vi "Simple TCP - Client.vi"() -> ()   [LabVIEW 2015]
doc: "Demonstrates how to open a connection to an TCP server, read the data being sent, and display the data on a chart. This VI is designed to stop if the TCP connection is terminated."
uses:
  <vilib>/Platform/TimedLoop/XDataNode/timing_clust.ctl
  <vilib>/Platform/TimedLoop/XDataNode/nitl_modes.ctl
  <vilib>/Platform/TimedLoop/XDataNode/wakeup.ctl
  <vilib>/platform/TimedLoop/XDataNode/XDataNode.xnode
  <vilib>/Platform/TimedLoop/XDataNode/XDNodeRunTimeDep.lvlib
panel:
  out "Counter":i32
  out "Time":u32
  out "value":T1
  in  "Server Closed":string="The server VI closed the connection."
  in  "Stop":bool
  # "Overview: Demonstrates the use of the TCP functions to connect to a TCP server VI and receive data.\nInstructions:\n1. Ensure Simple TCP - Server.vi is already running.\n2. Run the VI.\n3. Click Stop to stop the VI. Note that if you stop the server VI, this VI will stop automatically."
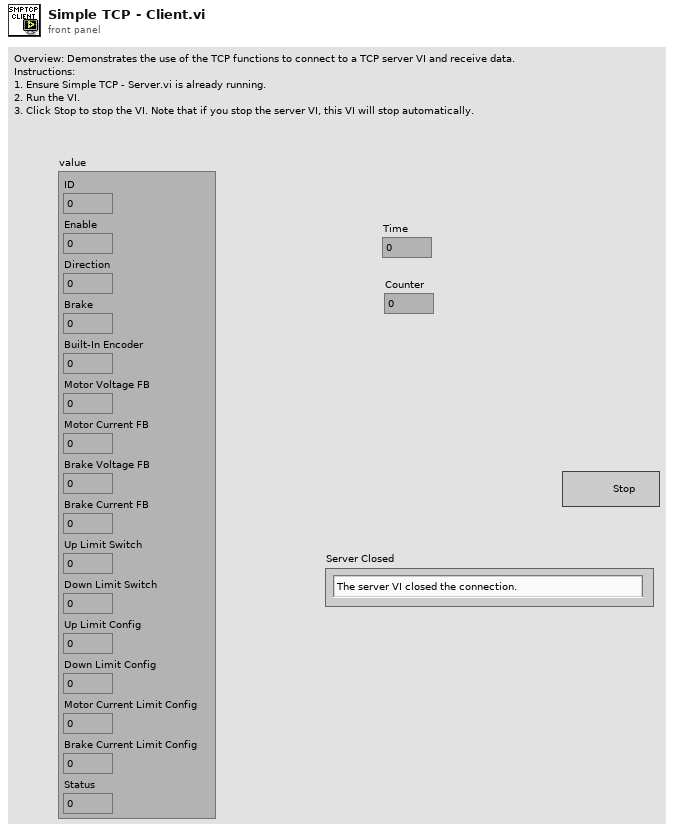
[diagram p1: front panel]
types:
  T1 = cluster{"ID":dbl, "Enable":dbl, "Direction":dbl, "Brake":dbl, "Built-In Encoder":dbl, "Motor Voltage FB":dbl, "Motor Current FB":dbl, "Brake Voltage FB":dbl, "Brake Current FB":dbl, "Up Limit Switch":dbl, "Down Limit Switch":dbl, "Up Limit Config":dbl, "Down Limit Config":dbl, "Motor Current Limit Config":dbl, "Brake Current Limit Config":dbl, "Status":dbl}
  T2 = typedef "XDNodeRunTimeDep.lvlib/timing_clust.ctl" = cluster{"Expected End [f-1]":u64, "Actual End [f-1]":u64, "Finished Late? [f-1]":bool, "Expected End [i-1]":u64, "Actual End [i-1]":u64, "Finished Late? [i-1]":bool, "Expected Start [i]":u64, "Actual Start [i]":u64, "Expected Start [f]":u64, "Actual Start [f]":u64, "Source Name":string, "Structure Name":string, "Period":i64, "Deadline":i64, "Offset":i64, "Start":i64, "Priority":i32, "Timeout":i32, "Mode":T3, "Wakeup Reason":T4, "Error":errorcluster, "Source Type":string, "Secondary Source Type":string, "Global End Time":u64, "Global Start Time":u64, "Frame Duration":u64, "Iteration Duration":u64, "Assigned CPU":i32, "I/O Scan Engine Mode":u32}
  T3 = typedef "XDNodeRunTimeDep.lvlib/nitl_modes.ctl" = enum32{"No Change", "Process missed periods, maintain original phase", "Discard missed periods, maintain original phase", "Process missed periods, ignore original phase", "Discard missed periods, ignore original phase"}
  T4 = typedef "XDNodeRunTimeDep.lvlib/wakeup.ctl" = enum32{"Normal", "Aborted", "Asynchronous wakeup", "Timing source error", "Timed loop error", "Timeout"}
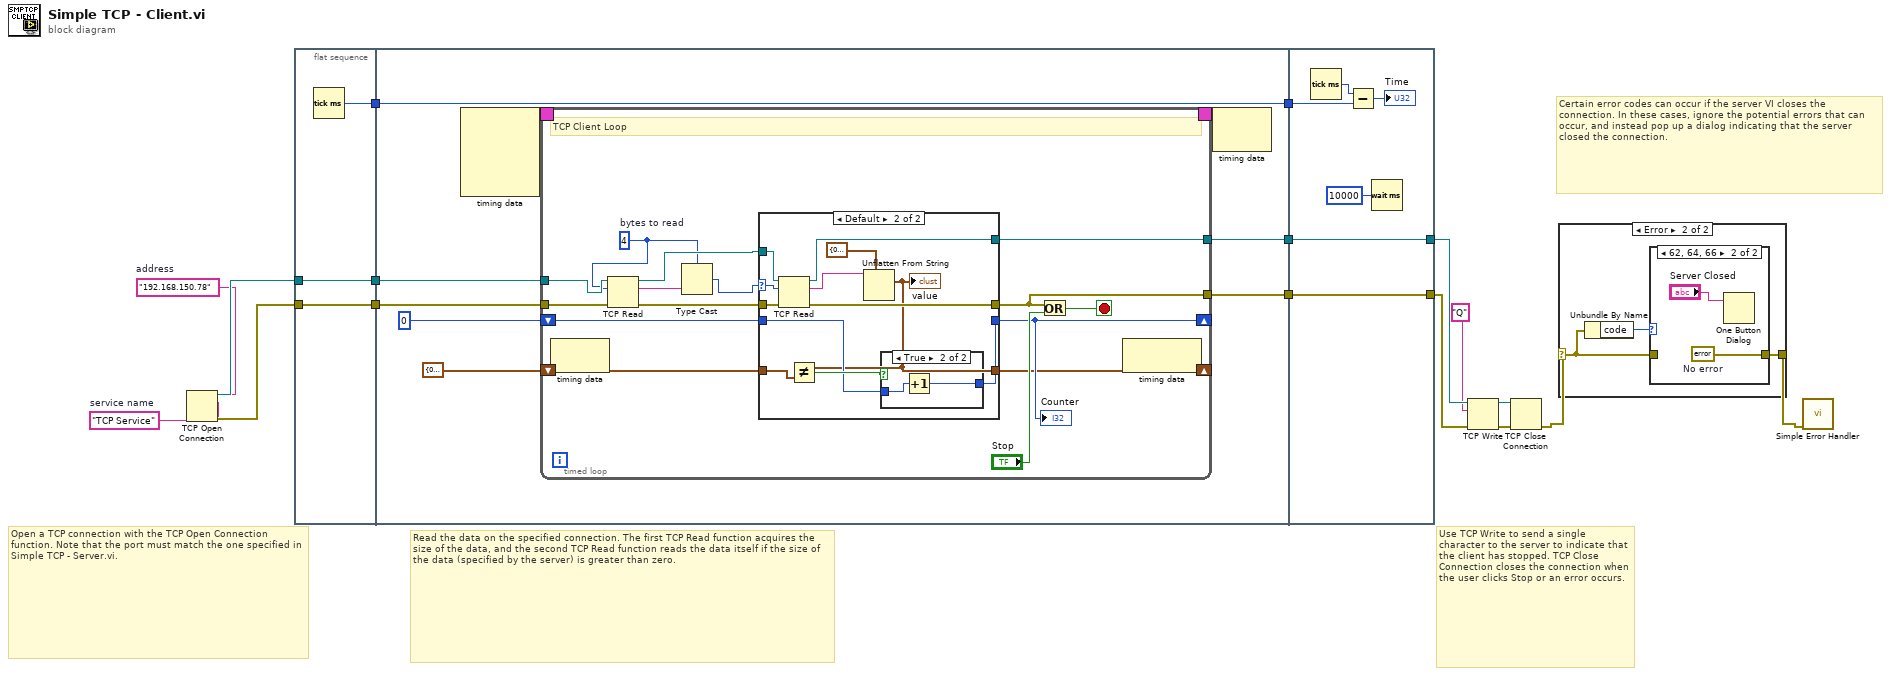
[diagram p0: block diagram]
diagram:
  w7 = "TCP Service"  # service name
  w8 = "192.168.150.78"  # address
  # "Certain error codes can occur if the server VI closes the connection. In these cases, ignore the potential errors that can occur, and instead pop up a dialog indicating that the server closed the connection."
  # "Use TCP Write to send a single character to the server to indicate that the client has stopped. TCP Close Connection closes the connection when the user clicks Stop or an error occurs."
  # "Read the data on the specified connection. The first TCP Read function acquires the size of the data, and the second TCP Read function reads the data itself if the size of the data (specified by the server) is greater than zero."
  # "Open a TCP connection with the TCP Open Connection function. Note that the port must match the one specified in Simple TCP - Server.vi."
  n1 = TCP Open Connection(address=w8, remote port or service name=w7) -> (connection ID=w17:refnum<k5>, error out=w16:errorcluster)  [unwired: 3 in]
  n2 = flat-sequence {
    tunnel: w16 -> [w19]
    tunnel: w17 -> [w20]
    tunnel: [w20] -> w6
    tunnel: [w19] -> w5
    tunnel: [w18] -> w1
    tunnel: w6 -> [w21]
    tunnel: w5 -> [w22]
    tunnel: [w27] -> w4
    tunnel: [w26] -> w3
    tunnel: [w23] -> w2
    tunnel: w1 -> [w23]
    tunnel: [w72] -> w12
    tunnel: [w73] -> w14
    tunnel: w4 -> [w73]
    tunnel: w3 -> [w72]
    tunnel: w2 -> [w70]
    frame #0 {
      n3 = Tick Count (ms)() -> (millisecond timer value=w18:u32)
    }
    frame #1 {
      n4 = node-c288() -> (w29:T2)  [unwired: 4 in]
      n5 = timed-loop {
        tunnel: [w42] -> w27
        tunnel: [w41] -> w26
        timing: w29 -> [_]
        timing-out: [_] -> w28
        shift-right: [w39] -> _
        shift-left: 0 -> [w40]
        shift-right: [w37] -> _
        shift-left: T1 {"ID"=0.0, "Enable"=0.0, "Direction"=0.0, "Brake"=0.0, "Built-In Encoder"=0.0, "Motor Voltage FB"=0.0, "Motor Current FB"=0.0, "Brake Voltage FB"=0.0, "Brake Current FB"=0.0, "Up Limit Switch"=0.0, "Down Limit Switch"=0.0, "Up Limit Config"=0.0, "Down Limit Config"=0.0, "Motor Current Limit Config"=0.0, "Brake Current Limit Config"=0.0, "Status"=0.0} ("MirrorCoverMotor") -> [w38]
        tunnel: w22 -> [w34]
        tunnel: w21 -> [w32]
        stop <- w43 stop-if-true
        w30 = 4  # bytes to read
        # "TCP Client Loop"
        n6 = node-c288() -> ()  [unwired: 1 in, 1 out]
        n7 = TCP Read(connection ID=w32, bytes to read=w30, error in (no error)=w34) -> (connection ID out=w33:refnum<k5>, data out=w35:string, error out=w31:errorcluster)  [unwired: 2 in]
        n8 = Type Cast(type=w30, x=w35) -> (*(type *) &x=w36:i32)
        n9 = case shown="Default" w36 {
          selector: w36 -> [_ w59]
          tunnel: w33 -> [w50 w62]
          tunnel: w31 -> [w47 w51]
          tunnel: [w50 w61] -> w42
          tunnel: [w47 w60] -> w41
          tunnel: w40 -> [w49 w54]
          tunnel: [w49 w53] -> w39
          tunnel: w38 -> [w48 w56]
          tunnel: [w48 w52] -> w37
          frame ..0 {
            # "The server has not written any data"
          }
          frame Default {
            n10 = TCP Read(connection ID=w62, bytes to read=w59, error in (no error)=w51) -> (connection ID out=w61:refnum<k5>, data out=w57:string, error out=w60:errorcluster)  [unwired: 2 in]
            n11 = Unflatten From String(type=T1 {"ID"=0.0, "Enable"=0.0, "Direction"=0.0, "Brake"=0.0, "Built-In Encoder"=0.0, "Motor Voltage FB"=0.0, "Motor Current FB"=0.0, "Brake Voltage FB"=0.0, "Brake Current FB"=0.0, "Up Limit Switch"=0.0, "Down Limit Switch"=0.0, "Up Limit Config"=0.0, "Down Limit Config"=0.0, "Motor Current Limit Config"=0.0, "Brake Current Limit Config"=0.0, "Status"=0.0} ("MirrorCoverMotor"), binary string=w57) -> (value=w52:T1)  [unwired: 3 in, 2 out]
            "value" <- w52
            n12 = Not Equal?(x=w52, y=w56) -> (x != y?=w55:bool)
            n13 = case shown="True" w55 {
              tunnel: w54 -> [w63 w65]
              tunnel: [w63 w64] -> w53
              frame False {
              }
              frame True {
                n14 = Increment(x=w65) -> (x+1=w64:i32)
              }
            }
          }
        }
        "Counter" <- w39
        n15 = Or(x=w41, y="Stop") -> (x .or. y?=w43:bool)
        n16 = node-c288() -> ()  [unwired: 1 in, 1 out]
      }
      n17 = node-c288(w28) -> ()  [unwired: 1 out]
    }
    frame #2 {
      n18 = Tick Count (ms)() -> (millisecond timer value=w71:u32)
      n19 = Subtract(x=w71, y=w70) -> (x-y=→"Time":u32)
      n20 = Wait (ms)(milliseconds to wait=u32 10000) -> ()  [unwired: 1 out]
    }
  }
  n21 = TCP Write(connection ID=w14, data in="Q", error in (no error)=w12) -> (connection ID out=w15:refnum<k5>, error out=w13:errorcluster)  [unwired: 2 out]
  n22 = TCP Close Connection(connection ID=w15, error in (no error)=w13) -> (error out=w10:errorcluster)  [unwired: 1 in, 1 out]
  n23 = case shown="Error" w10 {
    selector: w10 -> [w74 w76]
    tunnel: [w74 w75] -> w9
    frame No Error {
    }
    frame Error {
      n24 = Unbundle By Name(w76) -> ("code"=w77:i32)
      n25 = case shown="62, 64, 66" w77 {
        tunnel: w76 -> [w78 _]
        tunnel: [w78 w80] -> w75
        frame Default {
        }
        frame 62, 64, 66 {
          w80 = errorcluster {"status"=FALSE, "code"=0, "source"=""}  # No error
          n26 = One Button Dialog(message="Server Closed") -> ()  [unwired: 1 in, 1 out]
        }
      }
    }
  }
  n27 = call <vilib>:"Simple Error Handler.vi"("error in (no error)"=w9) -> ()  [unwired: 4 in, 5 out]
